vi "SEGUIDOR_DE_PAREDE.vi"(2 "NXT/EV3":T1) -> (0 "NXT/EV3 2":T1)   [LabVIEW 2016]
uses:
  <vilib>/NXT/Subs/LVHSConnector.ctl
  <vilib>/NXT/LegoClasses/BrickReference/BrickReference.lvclass
  <vilib>/NXT/Block Support/NXT_InputPort.ctl
  <vilib>/NXT/Block Support/NXT_OutputPort.ctl
  <vilib>/NXT/NXTIO Xnodes/NXTIONodeSubVIs/NXTMoveMotors.vi
  <vilib>/NXT/Dual Mode Library/Sensors/EV3_Ultrasonic_CM.vi
  <vilib>/NXT/Dual Mode Library/Sensors/Touch_Pressed.vi
  <vilib>/NXT/NXTIO Xnodes/AddressXNode/NXTIOAddress.xnode
  <vilib>/NXT/NXTIO Xnodes/NXTIOXNode/NXTIO.xnode
panel:
  in  "Kp":sgl
  in  "Dmin":sgl
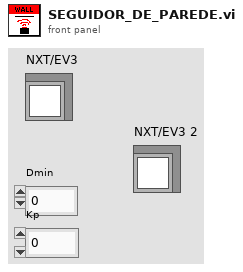
[diagram p1: front panel]
types:
  T1 = typedef "LVHSConnector.ctl" = refnum<class "BrickReference.lvclass">
  T2 = typedef "NXT_OutputPort.ctl" = u8
  T3 = typedef "NXT_InputPort.ctl" = u32
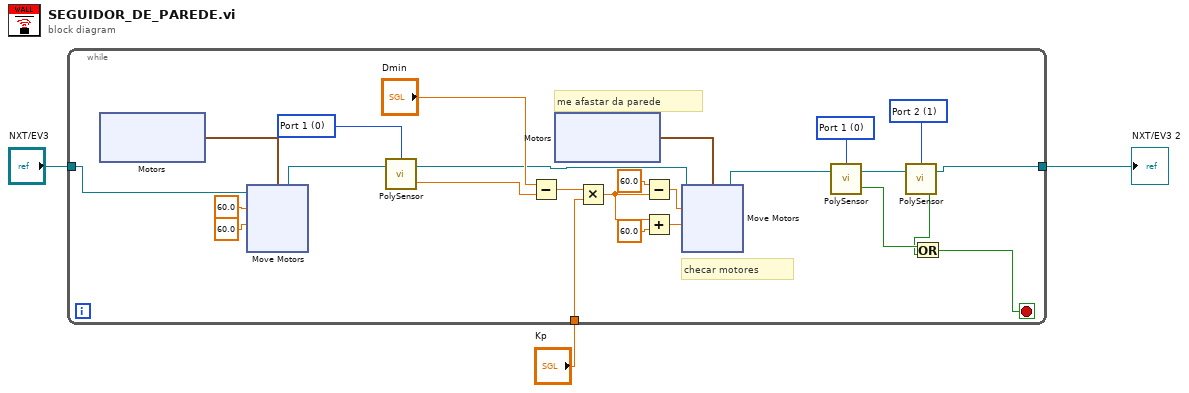
[diagram p0: block diagram]
diagram:
  n1 = while {
    tunnel: "NXT/EV3" -> [w22]
    tunnel: [w7] -> w2
    tunnel: "Kp" -> [w19]
    stop <- w4 stop-if-true
    w10 = T3 1 items=["Port 1", "Port 2", "Port 3", "Port 4"] ("Port (Port 1)")
    w9 = T3 0 items=["Port 1", "Port 2", "Port 3", "Port 4"] ("Port (Port 1)")
    w26 = T3 0 items=["Port 1", "Port 2", "Port 3", "Port 4"] ("Port (Port 1)")
    # "me afastar da parede"
    # "checar motores"
    n2 = xnode "Motors"() -> ("Motor"=w24:cluster{"Port":T2, "Port":T2})
    n3 = xnode "Move Motors"("Power/Speed 2"=sgl 60.0 ("x"), "Power/Speed 1"=sgl 60.0 ("x"), "Motors"=w24, "NXT/EV3"=w22) -> ("NXT/EV3"=w23:T1)
    n4 = call-poly <vilib>:"PolySensor.vi"("NXT/EV3"=w23, "Port (Port 1)"=w26) -> ("Centimeters"=w28:sgl, "NXT/EV3"=w25:T1)  [unwired: 1 in]
    n5 = Subtract(x="Dmin", y=w28) -> (x-y=w14:sgl)
    n6 = xnode "Motors"() -> ("Motor"=w15:cluster{"Port":T2, "Port":T2})
    n7 = Multiply(x=w14, y=w19) -> (x*y=w16:sgl)
    n8 = Subtract(x=sgl 60.0, y=w16) -> (x-y=w12:sgl)
    n9 = Add(x=w16, y=sgl 60.0 ("x")) -> (x+y=w13:sgl)
    n10 = xnode "Move Motors"("Power/Speed 2"=w13, "Power/Speed 1"=w12, "Motors"=w15, "NXT/EV3"=w25) -> ("NXT/EV3"=w8:T1)
    n11 = call-poly <vilib>:"PolySensor.vi"("NXT/EV3"=w8, "Port (Port 1)"=w9) -> ("Yes / No"=w6:bool, "NXT/EV3"=w11:T1)  [unwired: 1 in]
    n12 = call-poly <vilib>:"PolySensor.vi"("NXT/EV3"=w11, "Port (Port 1)"=w10) -> ("Yes / No"=w5:bool, "NXT/EV3"=w7:T1)  [unwired: 1 in]
    n13 = Or(x=w6, y=w5) -> (x .or. y?=w4:bool)
  }
  "NXT/EV3 2" <- w2
